vi "serial_comms.vi"() -> ()   [LabVIEW 2011]
uses:
  serial comms modes.ctl
  <vilib>/Instr/_visa.llb/VISA Configure Serial Port (Instr).vi
panel:
  in  "Port":refnum<visa-resource-name>
  in  "Mode":T1
  out "Error Out":errorcluster
  in  "Error In":errorcluster
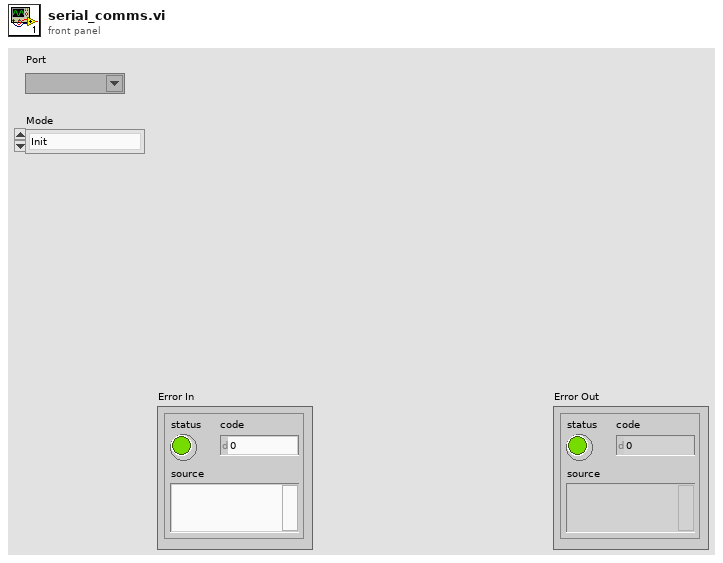
[diagram p1: front panel]
types:
  T1 = typedef "serial comms modes.ctl" = enum16{"Init", "Set/Get", "Close"}
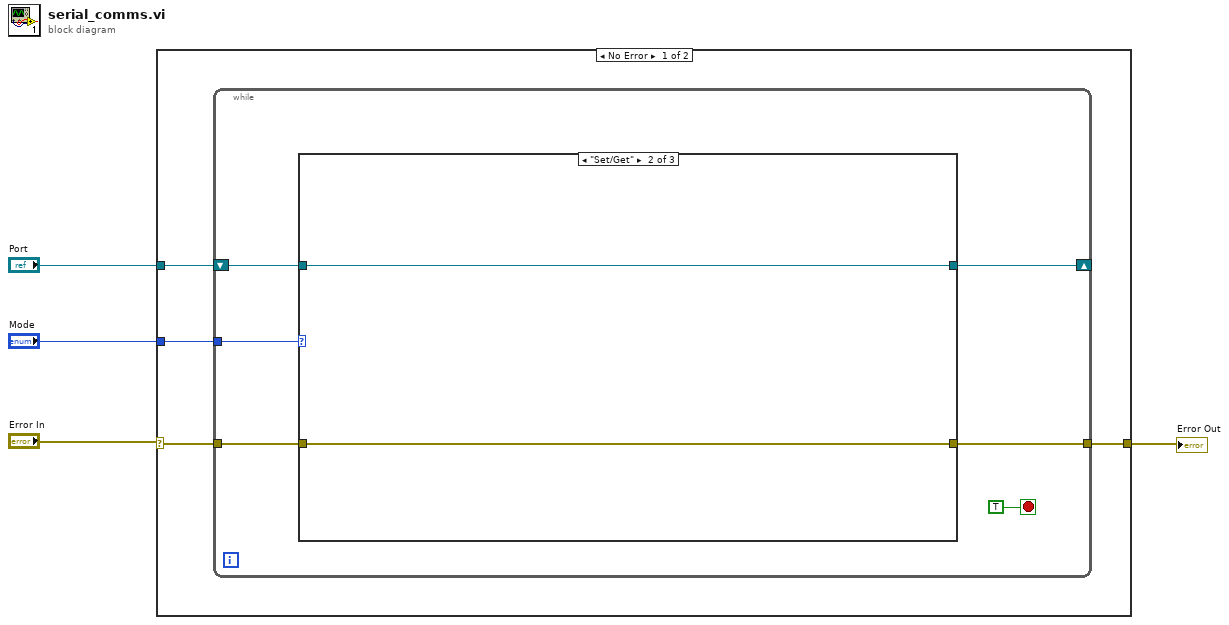
[diagram p0: block diagram]
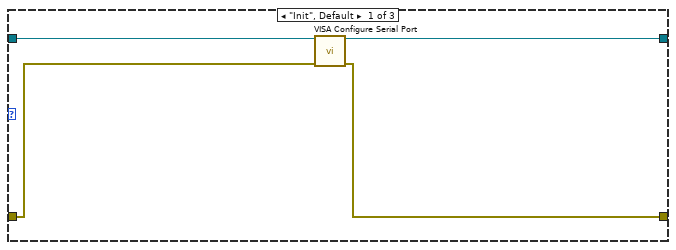
[diagram p2: hidden frame]
diagram:
  n1 = case shown="No Error" "Error In" {
    selector: "Error In" -> [w8 w23]
    tunnel: [w7 w23] -> w3
    tunnel: "Mode" -> [w6 _]
    tunnel: "Port" -> [w5 _]
    frame No Error {
      n2 = while {
        tunnel: w8 -> [w12]
        tunnel: [w11] -> w7
        tunnel: w6 -> [w13]
        shift-right: [w9] -> _
        shift-left: w5 -> [w10]
        stop <- TRUE stop-if-true
        n3 = case shown="\"Set/Get\"" w13 {
          tunnel: w12 -> [w17 w20 w22]
          tunnel: [w16 w20 w22] -> w11
          tunnel: w10 -> [w18 w19 w21]
          tunnel: [w15 w19 w21] -> w9
          frame "Init", Default {
            n4 = call-poly "VISA Configure Serial Port"("VISA resource name"=w18, "error in (no error)"=w17) -> ("VISA resource name out"=w15:refnum<visa-resource-name>, "error out"=w16:errorcluster)  [unwired: 12 in]
          }
          frame "Set/Get" {
          }
          frame "Close" {
          }
        }
      }
    }
    frame Error {
    }
  }
  "Error Out" <- w3
